vi "LocateFirstDerivativePeak.vi"(8 "error in (no error)":errorcluster, 11 "Graph":dbl[][](array[numeric])) -> (0 "error out":errorcluster, 3 "Ref":dbl)   [LabVIEW 2013, in "main.lvlib"]
uses:
  main.lvlib
  Controls/Enum Globals.ctl
  <vilib>/Analysis/NI_AALPro.lvlib
panel:
  out "System Waveform Graph 2":dbl[](graph)
  out "System Waveform Graph":dbl[](graph)
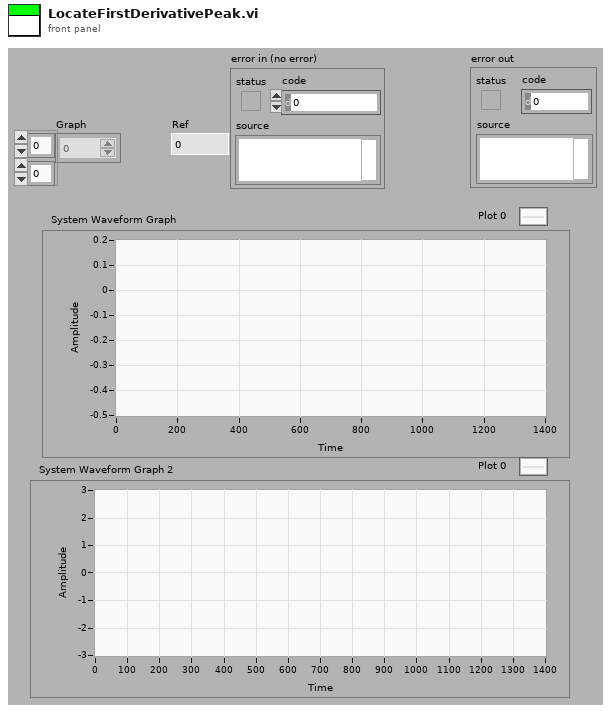
[diagram p1: front panel]
types:
  T1 = typedef "main.lvlib/Enum Globals.ctl" = enum16{"Init", "Set DataPath", "Set Freq", "Get"}
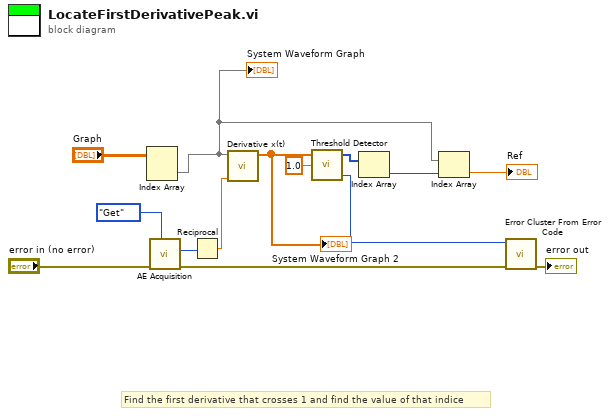
[diagram p0: block diagram]
diagram:
  # "Find the first derivative that crosses 1 and find the value of that indice"
  n1 = Index Array(array="Graph") -> (element=w7:dbl[])  [unwired: 2 in]
  "System Waveform Graph" <- w7
  n2 = call "AE Acquisition.vi"("Action"=Enum_Globals."Get", "error in (no error)"="error in (no error)") -> ("error out"=w2:errorcluster, "Freq Out"=w8:i32)  [unwired: 6 in, 2 out]
  n3 = Reciprocal(x=w8) -> (1/x=w12:dbl)
  n4 = call <vilib>:"Derivative x(t).vi"("dt"=w12, "X"=w7) -> ("dX/dt"=w5:dbl[])  [unwired: 8 in, 1 out]
  "System Waveform Graph 2" <- w5
  n5 = call <vilib>:"Threshold Detector.vi"("threshold"=1.0, "X"=w5) -> ("error"=w4:i32, "Indices"=w14:i32[])  [unwired: 1 in, 1 out]
  n6 = Index Array(array=w14) -> (element=w6:i32)  [unwired: 1 in]
  n7 = Index Array(array=w7, index=w6) -> (element=→"Ref":dbl)
  n8 = call <vilib>:"Error Cluster From Error Code.vi"("error in (no error)"=w2, "error code (0)"=w4) -> ("error out"=→"error out":errorcluster)  [unwired: 7 in]
